vi "Pass If In 1D Array (DBL).vi"(6 "expected index (optional)":i32=-1, 8 "error in (no error)":errorcluster, 9 "element":dbl, 10 "1D array":dbl[](array[numeric]), 11 "TestCase in":refnum<class "TestCase.lvclass">) -> (0 "error out":errorcluster, 3 "TestCase out":refnum<class "TestCase.lvclass">)   [LabVIEW 2015, in "VITAC.lvlib"]
doc: "Searches element in 1D DBL array, and returns pass if element is found. If <b>expected index (optional)</b> does not equal to -1, additionally compares found index with expected; and fails if they are not equal."
uses:
  VITAC.lvlib
  <vilib>/addons/_JKI Toolkits/VI Tester/TestCase.llb/TestCase.lvclass
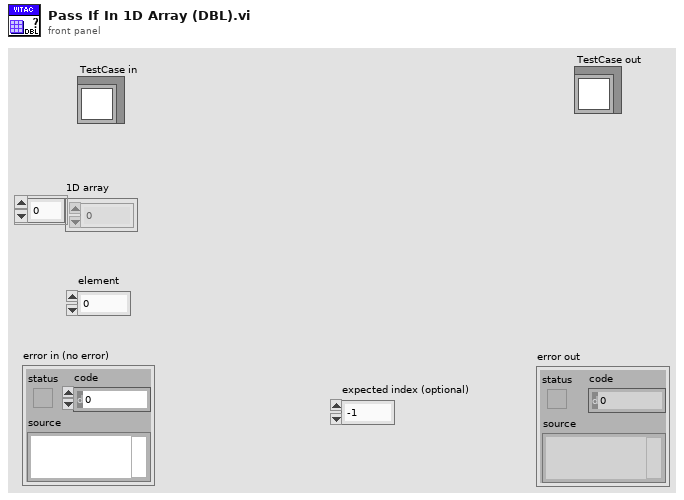
[diagram p1: front panel]
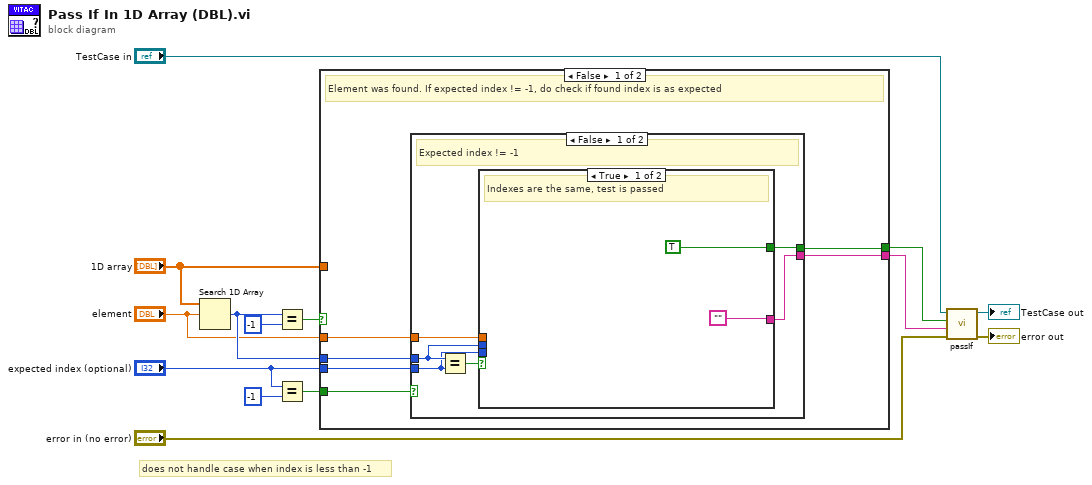
[diagram p0: block diagram]
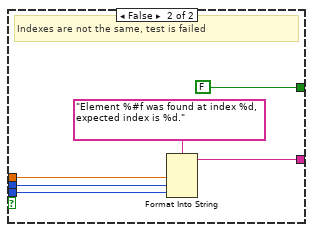
[diagram p2: hidden frame]
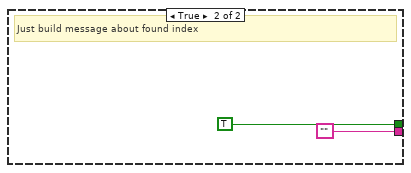
[diagram p3: hidden frame]
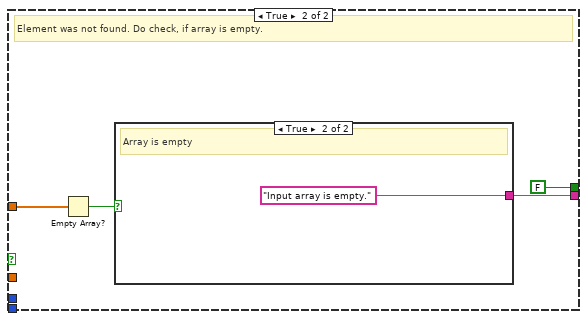
[diagram p4: hidden frame]
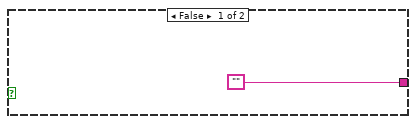
[diagram p5: hidden frame]
diagram:
  # "does not handle case when index is less than -1"
  n1 = Search 1D Array(1D array="1D array", element="element") -> (index of element=w5:i32)  [unwired: 1 in]
  n2 = Equal?(x=w5, y=-1) -> (x = y?=w8:bool)
  n3 = Equal?(x="expected index (optional)", y=-1) -> (x = y?=w2:bool)
  n4 = case shown="False" w8 {
    tunnel: "expected index (optional)" -> [w15 _]
    tunnel: [w19 FALSE] -> w10
    tunnel: [w16 w38] -> w9
    tunnel: "1D array" -> [_ w40]
    tunnel: w5 -> [w17 _]
    tunnel: w2 -> [w20 _]
    tunnel: "element" -> [w18 _]
    frame False {
      # "Element was found. If expected index != -1, do check if found index is as expected"
      n5 = case shown="False" w20 {
        tunnel: [w22 TRUE] -> w19
        tunnel: w18 -> [w25 _]
        tunnel: w17 -> [w24 _]
        tunnel: [w23 ""] -> w16
        tunnel: w15 -> [w21 _]
        frame False {
          # "Expected index != -1"
          n6 = Equal?(x=w24, y=w21) -> (x = y?=w26:bool)
          n7 = case shown="True" w26 {
            tunnel: w25 -> [_ w33]
            tunnel: w24 -> [_ w32]
            tunnel: ["" w31] -> w23
            tunnel: [TRUE FALSE] -> w22
            tunnel: w21 -> [_ w29]
            frame True {
              # "Indexes are the same, test is passed"
            }
            frame False {
              # "Indexes are not the same, test is failed"
              n8 = Format Into String(format string="Element %#f was found at index %d, expected index is %d.", w33, w32, w29) -> (resulting string=w31:string)  [unwired: 2 in, 1 out]
            }
          }
        }
        frame True {
          # "Just build message about found index"
        }
      }
    }
    frame True {
      # "Element was not found. Do check, if array is empty."
      n9 = Empty Array?(array=w40) -> (empty?=w39:bool)
      n10 = case shown="True" w39 {
        tunnel: ["" "Input array is empty."] -> w38
        frame False {
        }
        frame True {
          # "Array is empty"
        }
      }
    }
  }
  n11 = call-dynamic "passIf.vi"("error in (no error)"="error in (no error)", "message (\"\")"=w9, "pass"=w10, "TestCase in"="TestCase in") -> ("error out"=→"error out":errorcluster, "TestCase out"=→"TestCase out":refnum<class "TestCase.lvclass">)  [unwired: 6 in]
